vi "PWM Test - PDHydra PV.vi"() -> (0 "error out":errorcluster, 1 "RMS Values":dbl[](array[numeric]), 2 "DC Values":dbl[](array[numeric]), 3 "Frequency Values":dbl[](array[numeric]))   [LabVIEW 2022 SP3]
uses:
  HMP4000 Communication/HMP4040_ChannelControl.ctl
  <vilib>/DAQmx/read.llb/DAQmx Read (Analog 1D Wfm NChan NSamp).vi
  <vilib>/DAQmx/miscellaneous.llb/DAQmx Fill In Error Info.vi
panel:
  out "data":waveform(dbl)[](array[waveform])
  out "cluster":cluster{"data[0]":waveform(dbl)}
  in  "error in":errorcluster
  # "v"
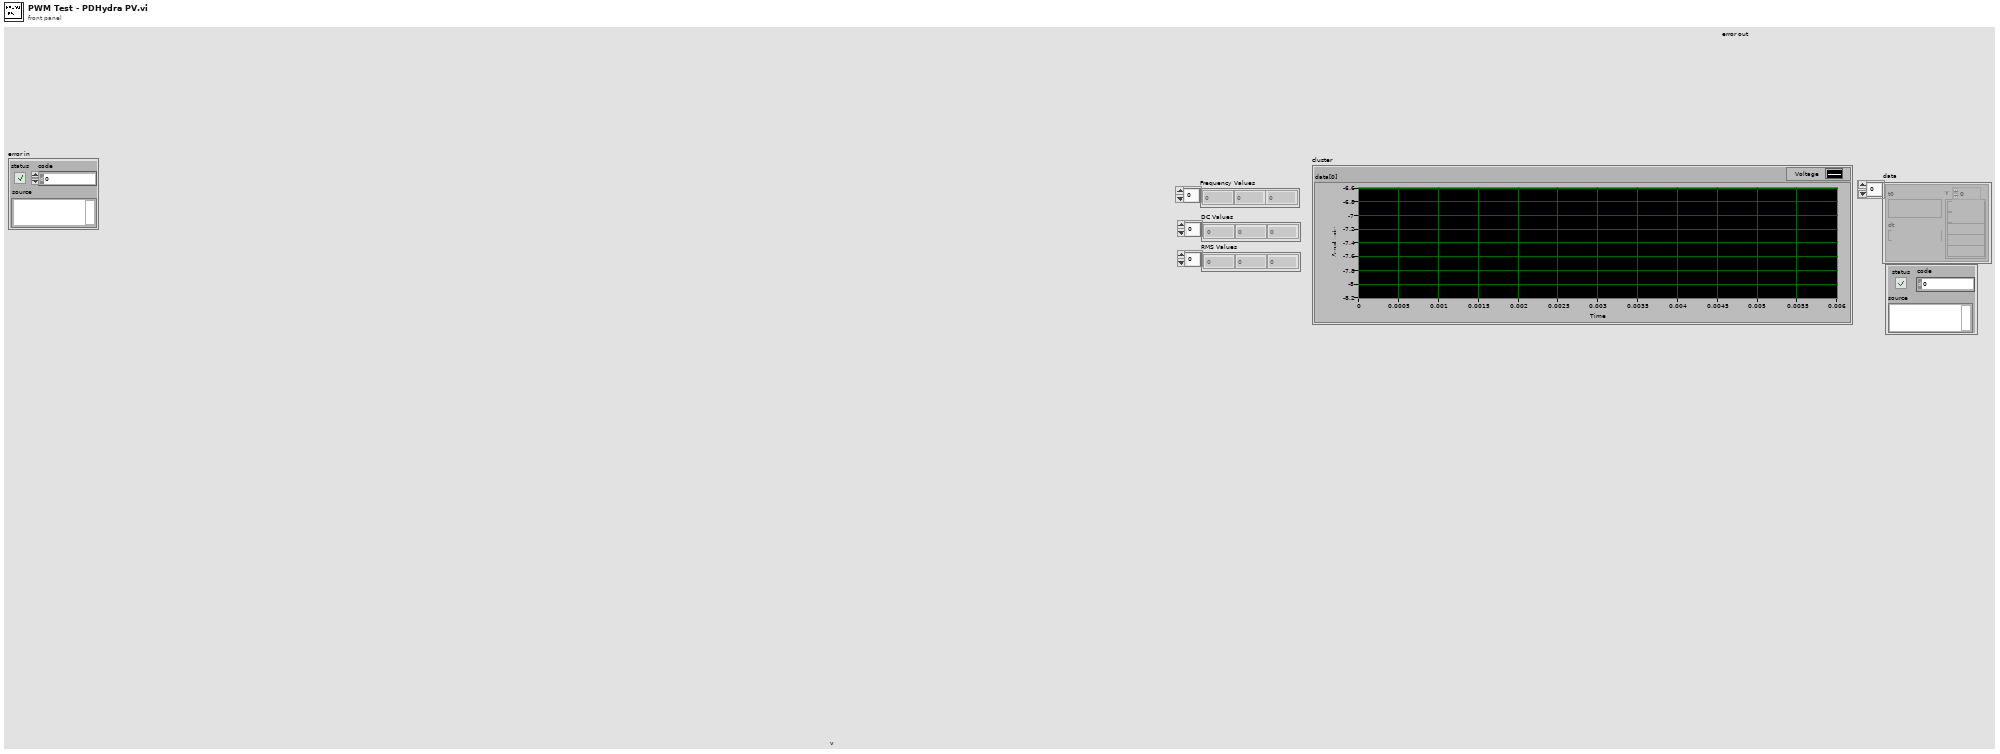
[diagram p1: front panel]
types:
  T1 = typedef "HMP4040_ChannelControl.ctl" = cluster{"CH1 Voltage":dbl, "CH1 Current":dbl, "CH1 Output":bool, "CH2 Voltage":dbl, "CH2 Current":dbl, "CH2 Output":bool, "CH3 Voltage":dbl, "CH3 Current":dbl, "CH3 Output":bool, "CH4 Voltage":dbl, "CH4 Current":dbl, "CH4 Output":bool, "Master Output":bool}
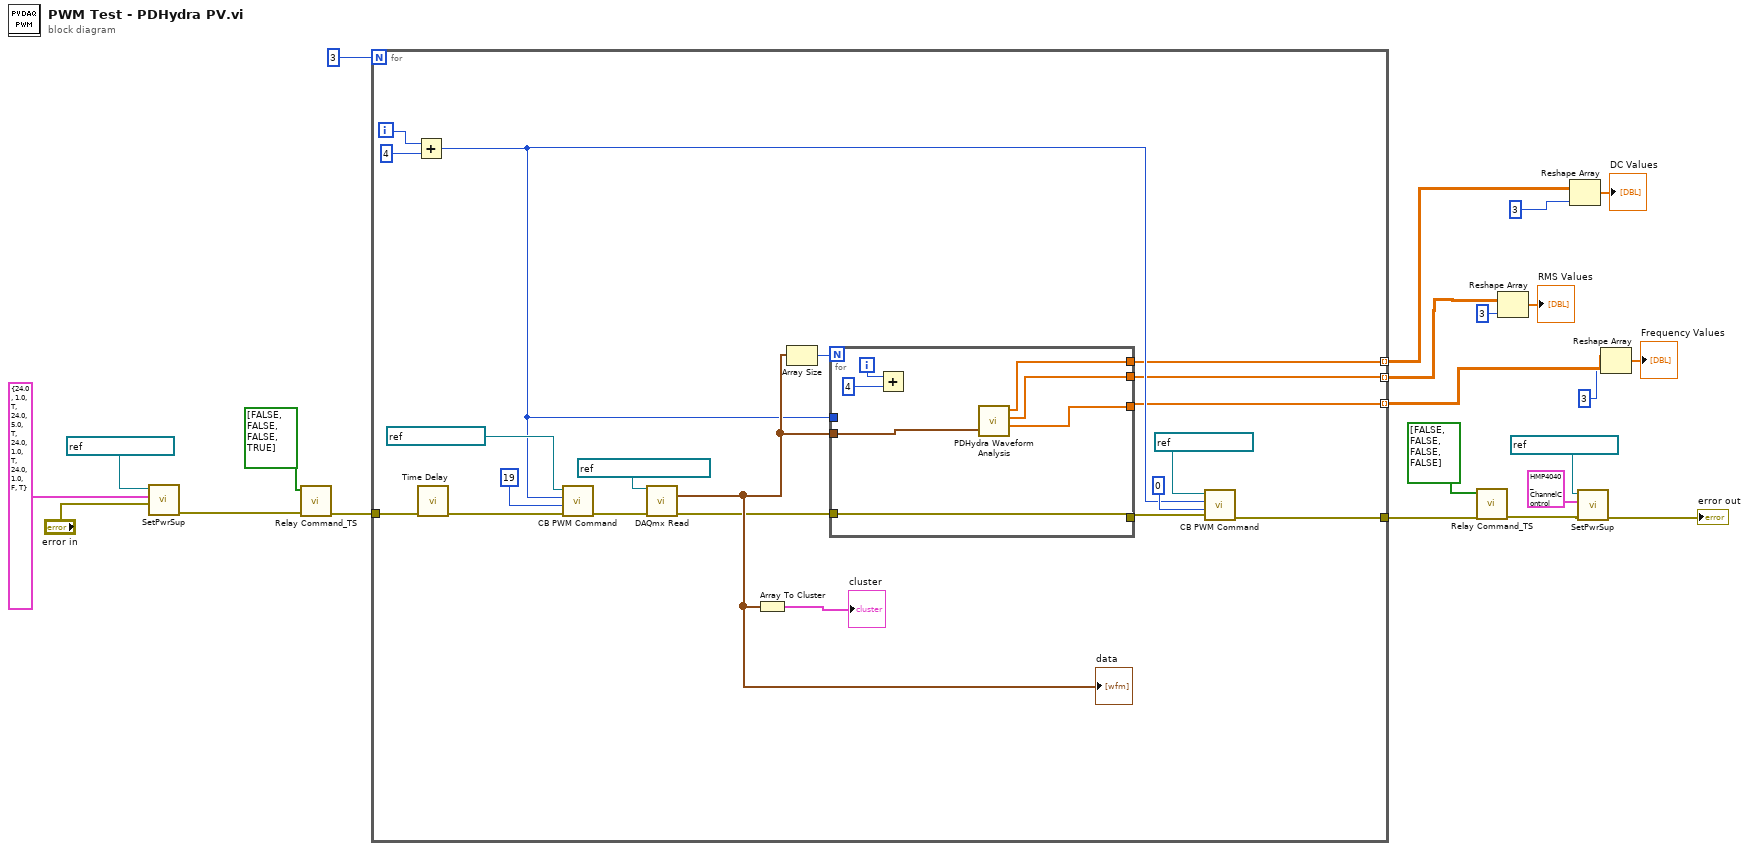
[diagram p0: block diagram]
diagram:
  n1 = call "SetPwrSup.vi"("error in (no error)"="error in", "HMP4040 Channel Settings"=T1 {"CH1 Voltage"=24.0, "CH1 Current"=1.0, "CH1 Output"=TRUE, "CH2 Voltage"=24.0, "CH2 Current"=5.0, "CH2 Output"=TRUE, "CH3 Voltage"=24.0, "CH3 Current"=1.0, "CH3 Output"=TRUE, "CH4 Voltage"=24.0, "CH4 Current"=1.0, "CH4 Output"=FALSE, "Master Output"=TRUE}, "HMP4040 IN"=refnum<visa-resource-name> "HMP4040_FTS2" ("VISA resource name")) -> ("error out"=w19:errorcluster)  [unwired: 7 in, 1 out]
  n2 = call "Relay Command_TS.vi"("error in (no error)"=w19, "Relay Command"=bool[] [FALSE, FALSE, FALSE, TRUE]) -> ("error out"=w17:errorcluster)  [unwired: 8 in, 1 out]
  n3 = for {
    N: 3 -> [_]
    tunnel: w17 -> [w38]
    tunnel: [w28] -> w15
    tunnel: [w25] -> w9 mode=indexing
    tunnel: [w24] -> w6 mode=indexing
    tunnel: [w23] -> w3 mode=indexing
    i -> [w27]
    n4 = Add(x=w27, y=4) -> (x+y=w31:i32)
    n5 = call "Time Delay"("error in (no error)"=w38) -> ("error out"=w37:errorcluster)  [unwired: 10 in]
    n6 = call "CB PWM Command.vi"("error in (no error)"=w37, "Duty Cycle"=19, "Leg"=w31, "VISA Refnum in"=refnum<visa-resource-name> "ControlBoard" ("Control Board In")) -> ("error out"=w40:errorcluster)  [unwired: 5 in, 2 out]
    n7 = call-poly <vilib>:"DAQmx Read.vi"("task/channels in"=refnum<k21> "FTS2_PWMInput_PV", "error in"=w40) -> ("data"=w34:waveform(dbl)[], "error out"=w29:errorcluster)  [unwired: 11 in, 1 out]
    "data" <- w34
    n8 = Array To Cluster(array=w34) -> (cluster=→"cluster":cluster{"data[0]":waveform(dbl)})
    n9 = Array Size(array=w34) -> (size(s)=w35:i32)
    n10 = for {
      N: w35 -> [_]
      tunnel: w34 -> [w45]
      tunnel: w31 -> [_]
      tunnel: [w48] -> w30
      tunnel: w29 -> [w48]
      tunnel: [w46] -> w25
      tunnel: [w44] -> w24
      tunnel: [w43] -> w23
      i -> [w47]
      n11 = Add(x=w47, y=4) -> ()  [unwired: 1 out]
      n12 = call "PDHydra Waveform Analysis.vi"("Waveform"=w45) -> ("Frequency"=w43:dbl[], "RMS values"=w44:dbl[], "DC values"=w46:dbl[])  [unwired: 8 in]
    }
    n13 = call "CB PWM Command.vi"("error in (no error)"=w30, "Duty Cycle"=0, "Leg"=w31, "VISA Refnum in"=refnum<visa-resource-name> "ControlBoard") -> ("error out"=w28:errorcluster)  [unwired: 5 in, 2 out]
  }
  n14 = call "Relay Command_TS.vi"("error in (no error)"=w15, "Relay Command"=bool[] [FALSE, FALSE, FALSE, FALSE]) -> ("error out"=w13:errorcluster)  [unwired: 8 in, 1 out]
  n15 = Reshape Array(w6, 3 ("dimension size")) -> (→"RMS Values":dbl[])
  n16 = Reshape Array(w9, 3 ("dimension size")) -> (→"DC Values":dbl[])
  n17 = call "SetPwrSup.vi"("error in (no error)"=w13, "HMP4040 Channel Settings"=T1 {"CH1 Voltage"=24.0, "CH1 Current"=1.0, "CH1 Output"=TRUE, "CH2 Voltage"=24.0, "CH2 Current"=5.0, "CH2 Output"=TRUE, "CH3 Voltage"=24.0, "CH3 Current"=1.0, "CH3 Output"=FALSE, "CH4 Voltage"=24.0, "CH4 Current"=1.0, "CH4 Output"=FALSE, "Master Output"=TRUE}, "HMP4040 IN"=refnum<visa-resource-name> "HMP4040_FTS2" ("VISA resource name")) -> ("error out"=→"error out":errorcluster)  [unwired: 7 in, 1 out]
  n18 = Reshape Array(w3, 3 ("dimension size")) -> (→"Frequency Values":dbl[])
